vi "AFG3352X.set phase.vi"(0 "i ref in":refnum<vi>, 1 "Channel (1: 1)":i32(ring)=1 items=["1"=1, "2"=2], 2 "Phase Angle (0 Degree)":dbl, 3 "ms timeout (10000)":i32=10000, 5 "error in (no error)":errorcluster) -> (14 "i ref out":refnum<vi>, 17 "timed out":bool, 19 "error out":errorcluster)   [LabVIEW 2014, in "AFG3352X.lvlib"]
doc: "Sets the amplitude at my device."
uses:
  AFG3352X.lvlib
  CS_Core/CSApplicationBaseClasses/AFGBase/AFGBase.serviceType.ctl
  CS_Core/CSApplicationBaseClasses/AFGBase/AFGBase.directionType.ctl
  CSlibraries/UtilityLib/UtilityLib.valueStatus.ctl
  CS_Core/CSApplicationBaseClasses/DeviceBase/DeviceBase.lvlib
  CS_Core/CSApplicationBaseClasses/AFGBase/AFGBase.lvlib
  CSlibraries/UtilityLib/UtilityLib.lvlib
  instr.lib/Agilent 3352X Series/Agilent 3352X Series.lvlib
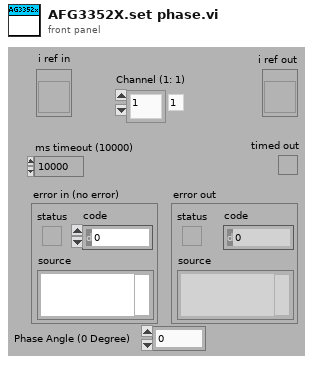
[diagram p1: front panel]
types:
  T1 = typedef "UtilityLib.lvlib/UtilityLib.valueStatus.ctl" = enum16{"no info available", "stand by/off", "on", "warning", "alarm/malfunction", "not implemented", "user action required", "important information", "system default", "control default", "indicator default", "button default"}
  T2 = typedef "AFGBase.lvlib/AFGBase.directionType.ctl" = enum16{"unknown", "update actual value", "update nominal value", "update both"}
  T3 = typedef "AFGBase.lvlib/AFGBase.serviceType.ctl" = enum16{"frequency", "amplitude", "phase", "DCOffset", "enableOutput", "trigger", "waveformType"}
  T4 = typedef "AFG3352X.lvlib/AFG3352X.i attribute.ctl" = cluster{"Act2ndValues":cluster{"frequency":dbl, "amplitude":dbl, "phase":dbl, "DCOffset":dbl, "waveformType":T5, "enableOutput":bool, "trigger":i16[], "serviceIDs":cluster{"frequencyID":i32, "amplitudeID":i32, "phaseID":i32, "DCOffsetID":i32, "waveformTypeID":i32, "enableOutputID":i32, "triggerID":i32}, "waveform":cluster{"data":waveform(dbl), "gain":dbl, "offset":dbl, "repetitionRate":dbl, "sampleRate":dbl}}, "Nom2ndValues":cluster{"frequency":dbl, "amplitude":dbl, "phase":dbl, "DCOffset":dbl, "waveformType":T5, "enableOutput":bool, "trigger":i16[], "serviceIDs":cluster{"frequencyID":i32, "amplitudeID":i32, "phaseID":i32, "DCOffsetID":i32, "waveformTypeID":i32, "enableOutputID":i32, "triggerID":i32}, "waveform":cluster{"data":waveform(dbl), "gain":dbl, "offset":dbl, "repetitionRate":dbl, "sampleRate":dbl}}, "DefaultChannel":i32, "ActAddValues":cluster{"Mode1":u16, "serviceIDs":cluster{"Mode1ID":i32, "Mode2ID":i32, "Burst1ID":i32, "Burst2ID":i32}, "Mode2":u16, "Burst1":i32, "Burst2":i32}, "NomAddValues":cluster{"Mode1":u16, "serviceIDs":cluster{"Mode1ID":i32, "Mode2ID":i32, "Burst1ID":i32, "Burst2ID":i32}, "Mode2 2":u16, "Burst1":i32, "Burst2":i32}, "enableBurstMode":bool}
  T5 = typedef "AFGBase.lvlib/AFGBase.waveformType.ctl" = enum16{"sine", "square", "ramp", "pulse", "noise", "DC", "arbitrary", "triangle", "ramp_up", "ramp_down", "amplitude modulation"}
  T6 = typedef "AFGBase.lvlib/AFGBase.i attribute.ctl" = cluster{"actValues":T7, "nomValues":T7}
  T7 = typedef "AFGBase.lvlib/AFGBase.parameters.ctl" = cluster{"frequency":dbl, "amplitude":dbl, "phase":dbl, "DCOffset":dbl, "waveformType":T5, "enableOutput":bool, "trigger":i16[], "serviceIDs":cluster{"frequencyID":i32, "amplitudeID":i32, "phaseID":i32, "DCOffsetID":i32, "waveformTypeID":i32, "enableOutputID":i32, "triggerID":i32}, "waveform":cluster{"data":waveform(dbl), "gain":dbl, "offset":dbl, "repetitionRate":dbl, "sampleRate":dbl}}
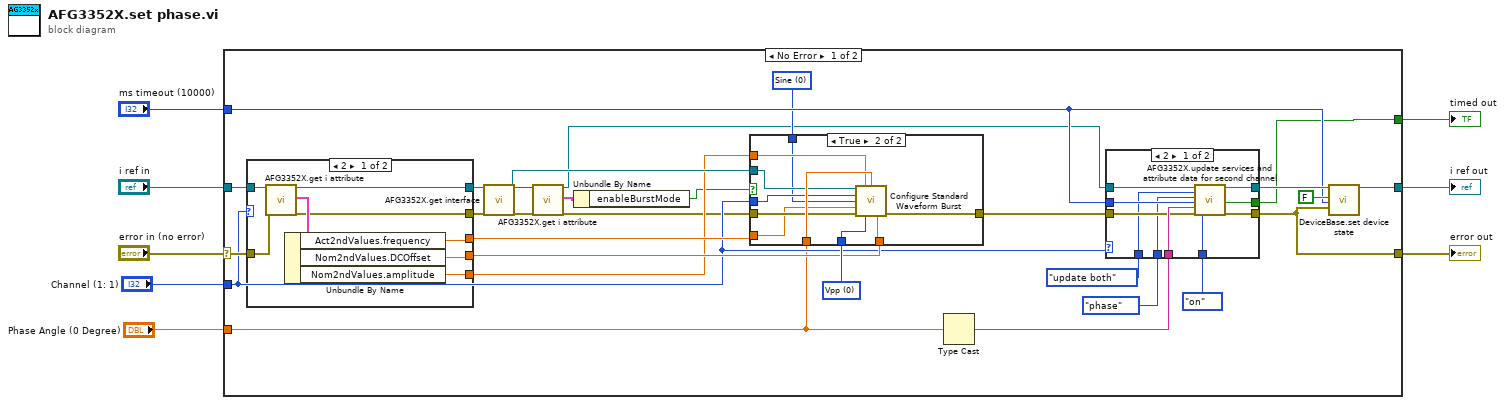
[diagram p0: block diagram]
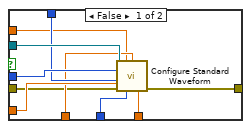
[diagram p2: hidden frame]
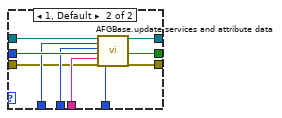
[diagram p3: hidden frame]
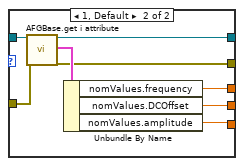
[diagram p4: hidden frame]
diagram:
  n1 = case shown="No Error" "error in (no error)" {
    selector: "error in (no error)" -> [w27 w94]
    tunnel: [w37 w95] -> w8
    tunnel: "ms timeout (10000)" -> [w33 _]
    tunnel: "i ref in" -> [w28 w95]
    tunnel: [w34 w94] -> w4
    tunnel: "Phase Angle (0 Degree)" -> [w16 _]
    tunnel: [w22 _] -> w3
    tunnel: "Channel (1: 1)" -> [w18 _]
    frame No Error {
      w17 = 0 items=["Sine"=0, "Square"=1, "Ramp"=2, "Noise"=3, "DC"=4, "Triangle"=5, "Pulse"=6, "Sinc"=11, "D-Lorentz"=12, "Gaussian"=13, "Expo Fall"=14, "Expo Rise"=15, "Haversine"=16] ("Waveform Function (0: Sine)")
      w21 = u16 0 items=["Vpp", "Vrms", "dB"] ("Unit (0: Vpp)")
      n2 = case shown="2" w18 {
        tunnel: w28 -> [w85 w93]
        tunnel: w27 -> [w82 w92]
        tunnel: [w84 w90] -> w26
        tunnel: [w81 w89] -> w25
        tunnel: [w79 w88] -> w20
        tunnel: [w80 w87] -> w19
        tunnel: [w78 w86] -> w15
        frame 2 {
          n3 = call "AFG3352X.get i attribute.vi"("i ref in"=w85, "error in (no error)"=w82) -> ("i ref out"=w84:refnum<vi>, "i attribute"=w83:T4, "error out"=w81:errorcluster)  [unwired: 15 in]
          n4 = Unbundle By Name(w83) -> ("Act2ndValues.frequency"=w79:dbl, "Nom2ndValues.DCOffset"=w80:dbl, "Nom2ndValues.amplitude"=w78:dbl)
        }
        frame 1, Default {
          n5 = call "AFGBase.get i attribute.vi"("i ref in"=w93, "error in (no error)"=w92) -> ("i ref out"=w90:refnum<vi>, "i attribute"=w91:T6, "error out"=w89:errorcluster)  [unwired: 15 in]
          n6 = Unbundle By Name(w91) -> ("nomValues.frequency"=w88:dbl, "nomValues.DCOffset"=w87:dbl, "nomValues.amplitude"=w86:dbl)
        }
      }
      n7 = call "AFG3352X.get interface.vi"("i ref in"=w26, "error in (no error)"=w25) -> ("i ref out"=w13:refnum<vi>, "interface"=w24:refnum<visa-resource-name>, "error out"=w11:errorcluster)  [unwired: 15 in]
      n8 = call "AFG3352X.get i attribute.vi"("i ref in"=w13, "error in (no error)"=w11) -> ("i ref out"=w12:refnum<vi>, "i attribute"=w14:T4, "error out"=w10:errorcluster)  [unwired: 15 in]
      n9 = Unbundle By Name(w14) -> ("enableBurstMode"=w9:bool)
      n10 = case shown="True" w9 {
        tunnel: w24 -> [w47 w52]
        tunnel: [w46 w57] -> w23
        tunnel: w21 -> [w45 w55]
        tunnel: w20 -> [w44 w49]
        tunnel: w19 -> [w43 w56]
        tunnel: w18 -> [w42 w51]
        tunnel: w17 -> [w41 w48]
        tunnel: w16 -> [w40 w54]
        tunnel: w15 -> [w39 w53]
        tunnel: w10 -> [w38 w50]
        frame False {
          n11 = call "Configure Standard Waveform.vi"("VISA resource name"=w47, "Amplitude (0.1 Vpp)"=w39, "Phase Angle (0 Degree)"=w40, "Channel (1: 1)"=w42, "Waveform Function (0: Sine)"=w41, "Frequency/Sample Rate/Bandwidth (1000 Hz)"=w44, "error in (no error)"=w38, "Amplitude Unit (0: Vpp)"=w45, "DC Offset (0 V)"=w43) -> ("error out"=w46:errorcluster)  [unwired: 5 in, 1 out]
        }
        frame True {
          n12 = call "Configure Standard Waveform Burst.vi"("VISA resource name"=w52, "Amplitude (0.1 Vpp)"=w53, "Phase Angle (0 Degree)"=w54, "Channel (1: 1)"=w51, "Waveform Function (0: Sine)"=w48, "Frequency/Sample Rate/Bandwidth (1000 Hz)"=w49, "error in (no error)"=w50, "Amplitude Unit (0: Vpp)"=w55, "DC Offset (0 V)"=w56) -> ("error out"=w57:errorcluster)  [unwired: 5 in, 1 out]
        }
      }
      n13 = Type Cast(x=w16) -> (*(type *) &x=w31:string)  [unwired: 1 in]
      n14 = case shown="2" w18 {
        tunnel: [w59 w77] -> w35
        tunnel: [w64 w76] -> w34
        tunnel: w33 -> [w63 w75]
        tunnel: AFGBase.serviceType."phase" ("service") -> [w62 w74]
        tunnel: w31 -> [w66 w73]
        tunnel: AFGBase.directionType."update both" ("direction") -> [w61 w72]
        tunnel: UtilityLib.valueStatus."on" ("quality") -> [w67 w71]
        tunnel: w23 -> [w65 w70]
        tunnel: w12 -> [w60 w69]
        tunnel: [w58 w68] -> w22
        frame 2 {
          n15 = call "AFG3352X.update services and attribute data for second channel.vi"("i ref in"=w60, "direction"=w61, "service"=w62, "ms timeout (10000)"=w63, "value"=w66, "error in (no error)"=w65, "quality"=w67) -> ("i ref out"=w59:refnum<vi>, "timed out"=w58:bool, "error out"=w64:errorcluster)  [unwired: 10 in]
        }
        frame 1, Default {
          n16 = call "AFGBase.update services and attribute data.vi"("i ref in"=w69, "direction"=w72, "service"=w74, "ms timeout (10000)"=w75, "value"=w73, "error in (no error)"=w70, "quality"=w71) -> ("i ref out"=w77:refnum<vi>, "timed out"=w68:bool, "error out"=w76:errorcluster)  [unwired: 10 in]
        }
      }
      n17 = call "DeviceBase.set device state.vi"("i ref in"=w35, "implicit"=FALSE, "ms timeout (10000)"=w33, "device error"=w34) -> ("i ref out"=w37:refnum<vi>)  [unwired: 13 in, 2 out]
    }
    frame Error {
    }
  }
  "error out" <- w4
  "i ref out" <- w8
  "timed out" <- w3
